vi "Debug_Convert_Data_to_String.vi"(8 "error in (no error)":errorcluster, 11 "AB_Source_RESTfulVI in":refnum<class "AB_Source_RESTfulVI.lvclass">) -> (0 "error out":errorcluster, 1 "classData":string, 2 "sourceType":string, 3 "AB_Source_RESTfulVI out":refnum<class "AB_Source_RESTfulVI.lvclass">)   [LabVIEW 2020, in "AB_Source_RESTfulVI.lvclass"]
uses:
  <vilib>/AppBuilder/AB_Classes/Source/RESTfulVI/AB_Source_RESTfulVI.lvclass
  <vilib>/AppBuilder/AB_Classes/Source/RESTfulVI/AB_Source_RESTfulVI.lvclass/AB_Source_RESTfulVI.ctl
  <vilib>/AppBuilder/AB_Classes/Source/VI/AB_Source_VI.lvclass
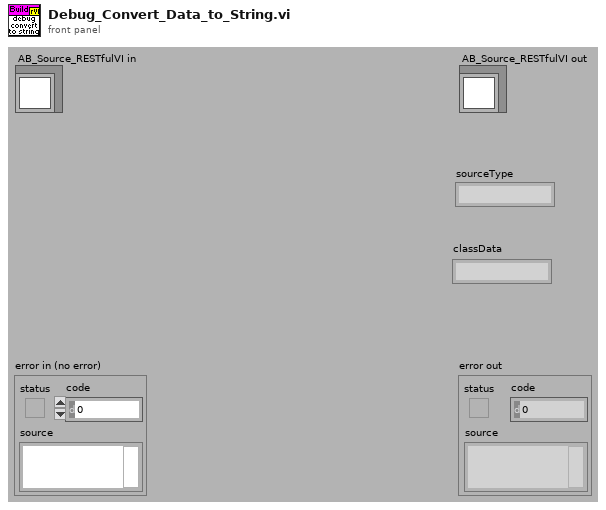
[diagram p1: front panel]
types:
  T1 = typedef "AB_RESTful_VIType.ctl" = enum32{"Web Method", "Auxiliary", "eng_Internal", "eng_Content"}
  T2 = typedef "AB_RESTful_OutputType.ctl" = enum32{"Terminal", "Stream"}
  T3 = typedef "AB_RESTful_OutputFormat.ctl" = enum32{"XML", "Text", "HTML", "JSON"}
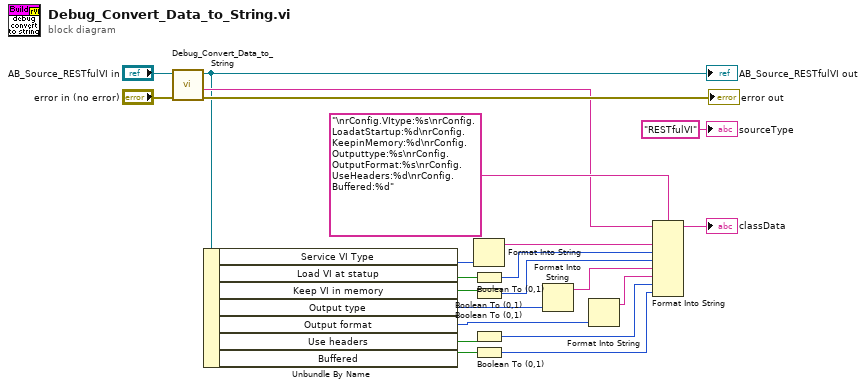
[diagram p0: block diagram]
diagram:
  n1 = call-parent "Debug_Convert_Data_to_String.vi"("error in (no error)"="error in (no error)", "AB_Source_VI in"="AB_Source_RESTfulVI in") -> ("error out"=→"error out":errorcluster, "classData"=w17:string, "AB_Source_VI out"=w15:refnum<class "AB_Source_RESTfulVI.lvclass">)  [unwired: 6 in, 1 out]
  "AB_Source_RESTfulVI out" <- w15
  n2 = Unbundle By Name(w15) -> ("Service VI Type"=w14:T1, "Load VI at statup"=w12:bool, "Keep VI in memory"=w11:bool, "Output type"=w2:T2, "Output format"=w4:T3, "Use headers"=w10:bool, "Buffered"=w9:bool)
  n3 = Format Into String(w14) -> (resulting string=w13:string)  [unwired: 3 in, 1 out]
  n4 = Boolean To (0,1)(Boolean=w12) -> (0, 1=w8:i16)
  n5 = Boolean To (0,1)(Boolean=w11) -> (0, 1=w7:i16)
  n6 = Boolean To (0,1)(Boolean=w10) -> (0, 1=w5:i16)
  n7 = Boolean To (0,1)(Boolean=w9) -> (0, 1=w6:i16)
  n8 = Format Into String(w2) -> (resulting string=w1:string)  [unwired: 3 in, 1 out]
  n9 = Format Into String(w4) -> (resulting string=w3:string)  [unwired: 3 in, 1 out]
  n10 = Format Into String(format string="\nrConfig.VItype:%s\nrConfig.LoadatStartup:%d\nrConfig.KeepinMemory:%d\nrConfig.Outputtype:%s\nrConfig.OutputFormat:%s\nrConfig.UseHeaders:%d\nrConfig.Buffered:%d", initial string=w17, w13, w8, w7, w1, w3, w5, w6) -> (resulting string=→"classData":string)  [unwired: 1 in, 1 out]
  "sourceType" <- "RESTfulVI" ("sourceType")
